vi "Read Root.vi"(8 "Error In":errorcluster, 11 "File In":refnum<class "File.lvclass">) -> (0 "Error Out":errorcluster, 2 "Root":path, 3 "File Out":refnum<class "File.lvclass">)   [LabVIEW 2018, in "Toolkit.lvlib" / "Loaders.lvlib" / "File.lvclass"]
uses:
  File.lvclass
  File.lvclass/File.ctl
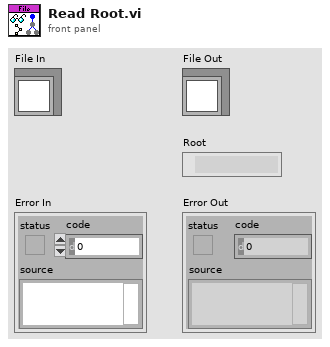
[diagram p1: front panel]
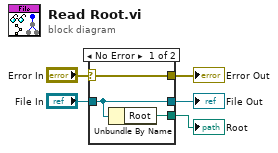
[diagram p0: block diagram]
diagram:
  n1 = case shown="No Error" "Error In" {
    selector: "Error In" -> [w8 w9]
    tunnel: [w8 w9] -> w4
    tunnel: [w7 w10] -> w2
    tunnel: "File In" -> [w7 w10]
    tunnel: [w6 _] -> w1
    frame No Error {
      n2 = Unbundle By Name(w7) -> ("Root"=w6:path)
    }
    frame Error {
    }
  }
  "Error Out" <- w4
  "File Out" <- w2
  "Root" <- w1
